vi "Untitled 71.vi"() -> ()   [LabVIEW 2017]
uses:
  <vilib>/addons/_office/excel.llb/Excel Easy Table (str).vi
  <vilib>/addons/_office/NI_ReportGenerationToolkit.lvlib
  <vilib>/Utility/NIReport.llb/NI_report.lvclass
panel:
  in  "Slide":dbl(slide) scale=0.0..4096.0
  # "V"
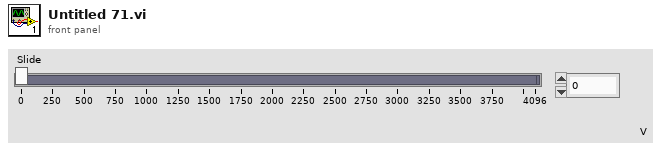
[diagram p1: front panel]
types:
  T1 = enum16{"Standard Report", "HTML", "Word", "Excel"}
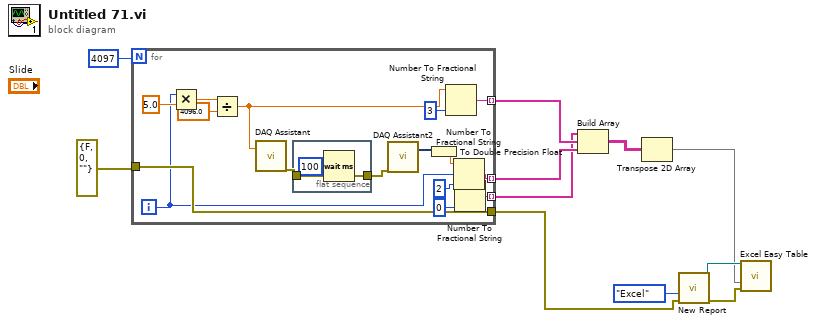
[diagram p0: block diagram]
diagram:
  n1 = for {
    N: 4097 -> [_]
    tunnel: [w24] -> w5
    tunnel: errorcluster {"status"=FALSE, "code"=0, "source"=""} ("error constant") -> [w24]
    tunnel: [w17] -> w3 mode=indexing
    tunnel: [w16] -> w2 mode=indexing
    tunnel: [w12] -> w1 mode=indexing
    i -> [w13]
    n2 = Multiply(x=w13, y=5.0) -> (x*y=w27:dbl)
    n3 = Divide(x=w27, y=4096.0) -> (x/y=w19:dbl)
    n4 = call "DAQ Assistant"("data"=w19) -> ("error out"=w23:errorcluster)  [unwired: 17 in, 1 out]
    n5 = flat-sequence {
      tunnel: w23 -> [w29]
      tunnel: [w29] -> w22
      frame #0 {
        n6 = Wait (ms)(milliseconds to wait=u32 100) -> ()  [unwired: 1 out]
      }
    }
    n7 = call "DAQ Assistant2"("error in"=w22) -> ("data"=w21:dynamicdata)  [unwired: 16 in, 2 out]
    n8 = To Double Precision Float(number=w21) -> (double precision float=w20:dbl)
    n9 = Number To Fractional String(number=w19, precision (6)=i16 3) -> (F-format string=w17:string)  [unwired: 2 in]
    n10 = Number To Fractional String(number=w20, precision (6)=i16 2) -> (F-format string=w16:string)  [unwired: 2 in]
    n11 = Number To Fractional String(number=w13, precision (6)=i16 0) -> (F-format string=w12:string)  [unwired: 2 in]
  }
  n12 = Build Array(w1, w3, w2) -> (w8:string[][])
  n13 = Transpose 2D Array(2D array=w8) -> (transposed array=w7:string[][])
  n14 = call <vilib>:"New Report.vi"("report type"=T1."Excel", "error in (no error)"=w5) -> ("report out"=w11:refnum<class "NI_report.lvclass">, "error out"=w6:errorcluster)  [unwired: 12 in]
  n15 = call-poly <vilib>:"Excel Easy Table.vi"("report in"=w11, "text data"=w7, "error in (no error)"=w6) -> ()  [unwired: 8 in, 5 out]
